vi "FGV for song.vi"(10 "mode":bool, 11 "write song":enum16{"0", "1"}(ring)) -> (3 "read song":enum16{"0", "1"}(ring))   [LabVIEW 2023]
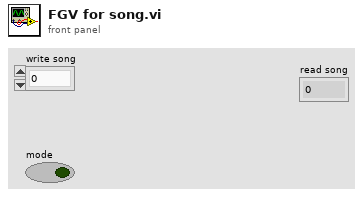
[diagram p1: front panel]
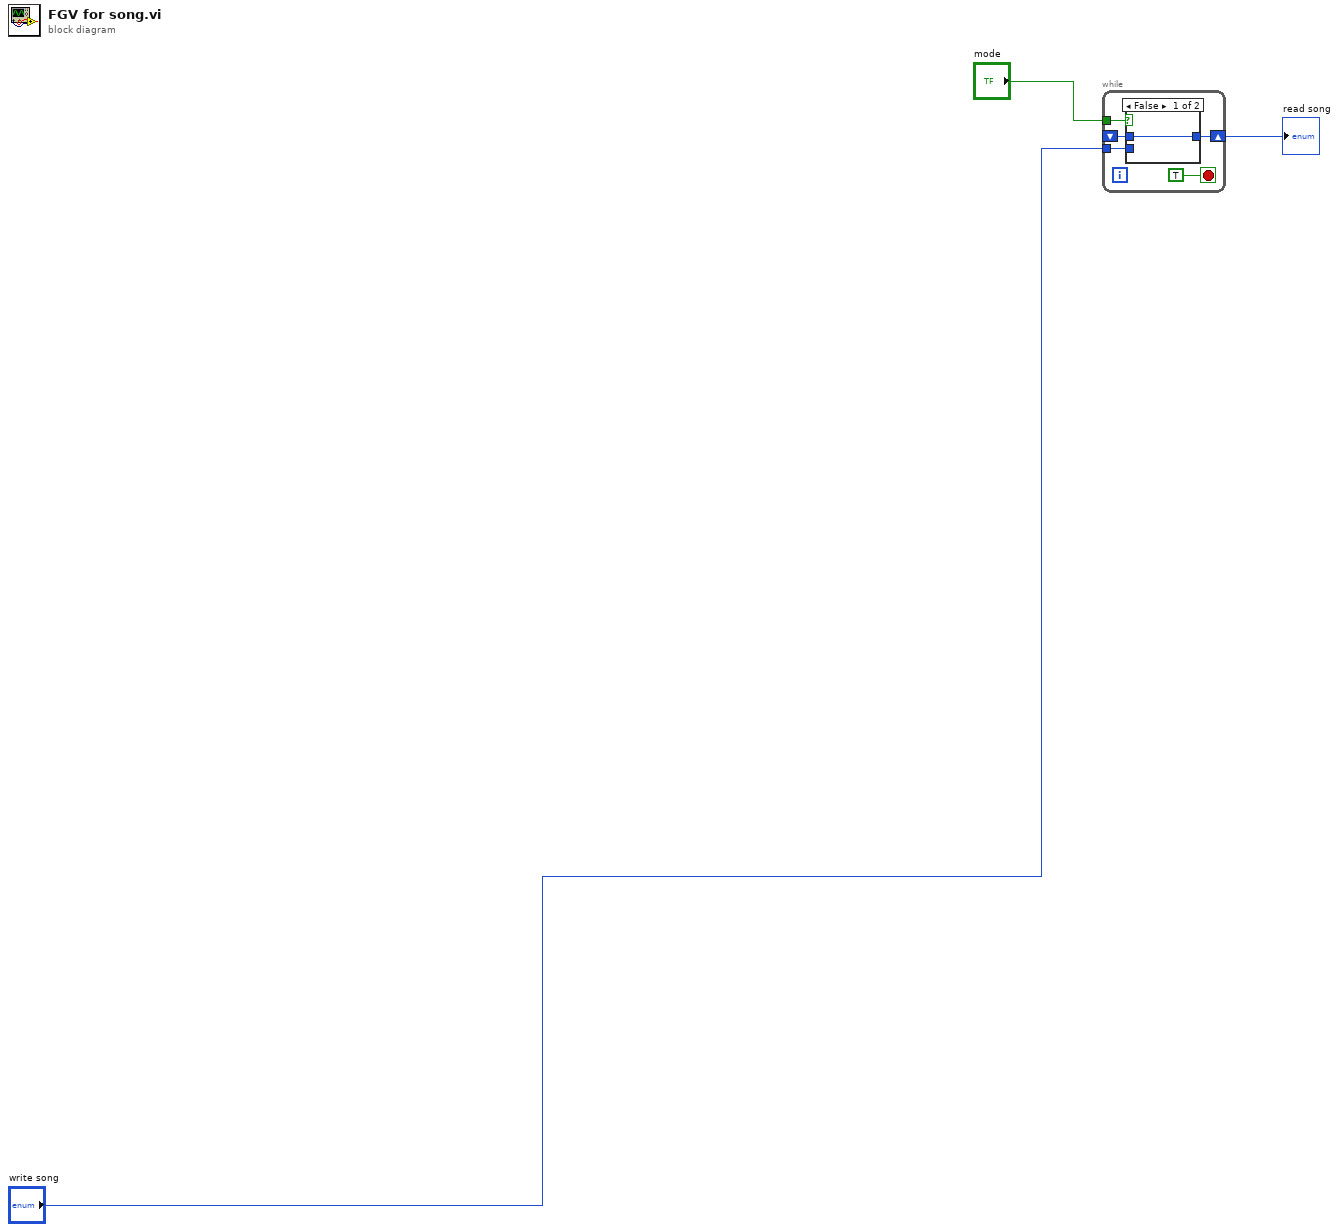
[diagram p0: block diagram]
diagram:
  n1 = while {
    tunnel: "write song" -> [w7]
    tunnel: "mode" -> [w8]
    shift-right: [w6] -> w1
    shift-left: _ -> [w5]
    stop <- TRUE stop-if-true
    n2 = case shown="False" w8 {
      tunnel: w7 -> [_ w10]
      tunnel: [w9 w10] -> w6
      tunnel: w5 -> [w9 _]
      frame False {
      }
      frame True {
      }
    }
  }
  "read song" <- w1
